vi "GoAndKickRoleVSS.vi"(7 "First call?":bool=TRUE, 8 "error in (no error)":errorcluster, 9 "Game in":refnum<class "Game.lvclass">, 11 "GoAndKickRoleVSS in":refnum<class "GoAndKickRoleVSS.lvclass">) -> (0 "error out":errorcluster, 1 "Game out":refnum<class "Game.lvclass">, 2 "Robot out":refnum<class "Robot.lvclass">, 3 "GoAndKickRoleVSS out":refnum<class "GoAndKickRoleVSS.lvclass">)   [LabVIEW 2023, in "GoAndKickRoleVSS.lvclass"]
uses:
  GoAndKickRoleVSS.lvclass
  Robot_class/Robot.lvclass
  Game_class/Game.lvclass
  Role_class/Role.lvclass/Role.ctl
  Role_class/Read Tacticbook.vi
  Role_class/Read tactic_index.vi
  Role_class/Write Tacticbook.vi
  Role_class/Write tactic_index.vi
  Role_class/Read RobotRef.vi
  Tacticbook_class/Tacticbook.lvclass
  DispBallTacticVSS_class/DispBallTacticVSS.lvclass
  DefendGoalTacticVSS_class/DefendGoalTacticVSS.lvclass
  PenaltyAttackTacticVSS_class/PenaltyAttackTacticVSS.lvclass
  DefendAreaTacticVSS_class/DefendAreaTacticVSS.lvclass
  AttackTacticVSS_class/AttackTacticVSS.lvclass
  HaltTactic_class/HaltTactic.lvclass
  GoAndKickTacticVSS_class/GoAndKickTacticVSS.lvclass
  GoalKickKeeperTacticVSS_class/GoalKickKeeperTacticVSS.lvclass
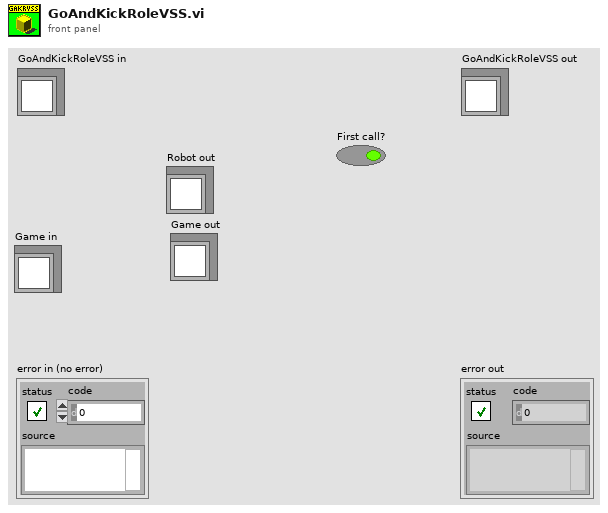
[diagram p1: front panel]
types:
  T1 = cluster{"DispBallTacticVSS":refnum<class "DispBallTacticVSS.lvclass">, "DefendGoalTacticVSS":refnum<class "DefendGoalTacticVSS.lvclass">, "PenaltyAttackTacticVSS":refnum<class "PenaltyAttackTacticVSS.lvclass">, "DefendAreaTacticVSS":refnum<class "DefendAreaTacticVSS.lvclass">, "AttackTacticVSS":refnum<class "AttackTacticVSS.lvclass">, "HaltTactic":refnum<class "HaltTactic.lvclass">, "GoAndKickTacticVSS":refnum<class "GoAndKickTacticVSS.lvclass">, "GoalKickKeeperTacticVSS":refnum<class "GoalKickKeeperTacticVSS.lvclass">}
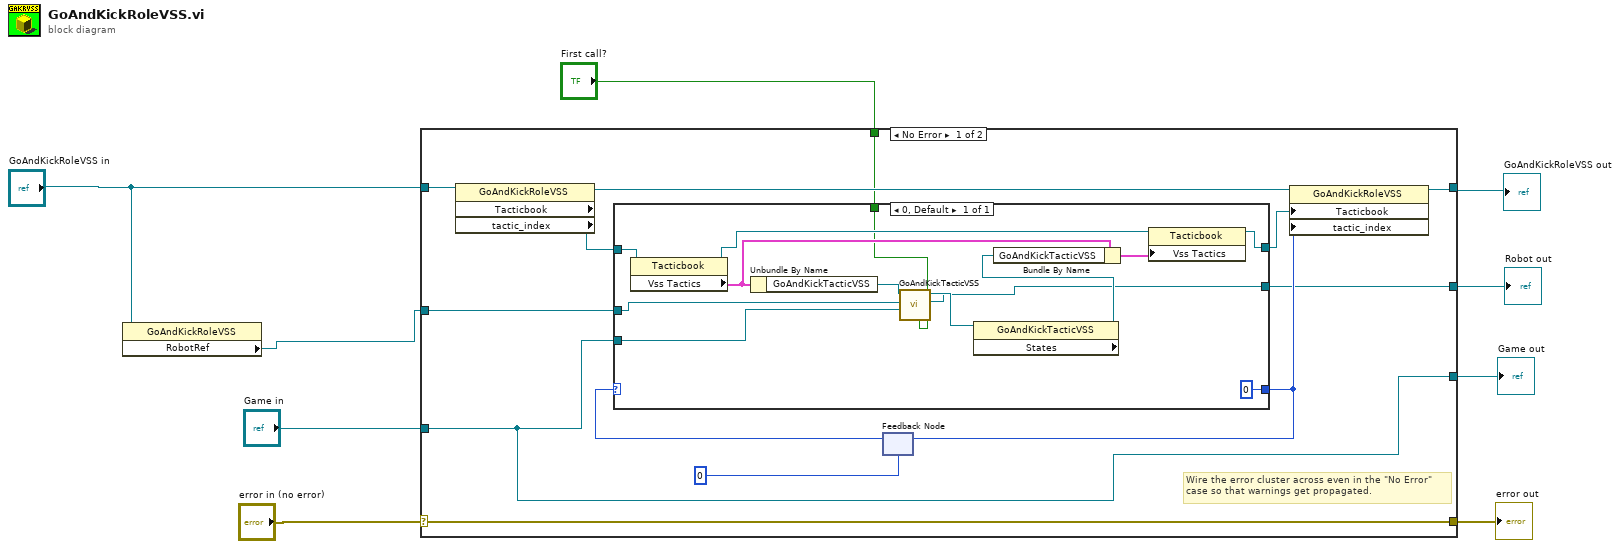
[diagram p0: block diagram]
diagram:
  n1 = property class="GoAndKickRoleVSS"(reference="GoAndKickRoleVSS in") -> ("RobotRef"=w9:refnum<class "Robot.lvclass">)  [unwired: 1 in, 2 out]
  n2 = case shown="No Error" "error in (no error)" {
    selector: "error in (no error)" -> [w22 w39]
    tunnel: [w22 w39] -> w7
    tunnel: [w20 w38] -> w4
    tunnel: "GoAndKickRoleVSS in" -> [w21 w38]
    tunnel: w9 -> [w14 w37]
    tunnel: [w13 w37] -> w5
    tunnel: [w11 w36] -> w6
    tunnel: "Game in" -> [w11 w36]
    tunnel: "First call?" -> [w10 _]
    frame No Error {
      # "Wire the error cluster across even in the \"No Error\"\ncase so that warnings get propagated."
      n3 = property class="GoAndKickRoleVSS" props=["Tacticbook", "tactic_index"](reference=w21) -> (reference out=w19:refnum<class "GoAndKickRoleVSS.lvclass">, "Tacticbook"=w16:refnum<class "Tacticbook.lvclass">)  [unwired: 1 in, 2 out]
      n4 = feedback #1(0) -> (w17:i32)
      n5 = case shown="0, Default" w17 {
        tunnel: [0] -> w15
        tunnel: w16 -> [w35]
        tunnel: w14 -> [w27]
        tunnel: [w23] -> w13
        tunnel: [w33] -> w12
        tunnel: w11 -> [w28]
        tunnel: w10 -> [w25]
        frame 0, Default {
          n6 = property class="Tacticbook"(reference=w35) -> (reference out=w34:refnum<class "Tacticbook.lvclass">, "Vss Tactics"=w31:T1)  [unwired: 1 in, 1 out]
          n7 = Unbundle By Name(w31) -> ("GoAndKickTacticVSS"=w26:refnum<class "GoAndKickTacticVSS.lvclass">)
          n8 = call "GoAndKickTacticVSS.vi"("First call?"=w25, "Game in"=w28, "Robot"=w27, "GoAndKickTacticVSS in"=w26) -> ("Robot out"=w23:refnum<class "Robot.lvclass">, "GoAndKickTacticVSS out"=w24:refnum<class "GoAndKickTacticVSS.lvclass">)  [unwired: 4 in, 2 out]
          n9 = property class="GoAndKickTacticVSS" props=["States"](reference=w24) -> (reference out=w29:refnum<class "GoAndKickTacticVSS.lvclass">)  [unwired: 1 in, 2 out]
          n10 = Bundle By Name(cluster=w31, "GoAndKickTacticVSS"=w29) -> (w30:T1)
          n11 = property class="Tacticbook"(reference=w34, "Vss Tactics"=w30) -> (reference out=w33:refnum<class "Tacticbook.lvclass">)  [unwired: 1 in, 1 out]
        }
      }
      n12 = feedback-in #1(w15) -> ()
      n13 = property class="GoAndKickRoleVSS"(reference=w19, "Tacticbook"=w12, "tactic_index"=w15) -> (reference out=w20:refnum<class "GoAndKickRoleVSS.lvclass">)  [unwired: 1 in, 1 out]
    }
    frame Error {
    }
  }
  "error out" <- w7
  "GoAndKickRoleVSS out" <- w4
  "Game out" <- w6
  "Robot out" <- w5
